vi "Overlay Pattern Matching Results #.vi"(7 "Group":string, 8 "error in":errorcluster, 9 "Result(PM)":cluster{"Name":string, "NG?":bool, "Score":dbl}, 10 "Matches":T2(array[cluster]), 11 "Image":T1) -> (0 "error out":errorcluster, 3 "Image Out":T1)   [LabVIEW 2013]
uses:
  <vilib>/vision/Image Controls.llb/IMAQ Image.ctl
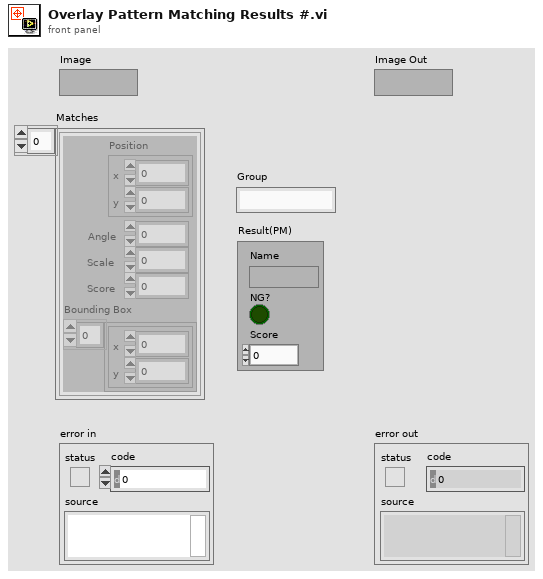
[diagram p1: front panel]
types:
  T1 = typedef "IMAQ Image.ctl" = refnum<image>
  T2 = cluster{"Position":cluster{"x":sgl, "y":sgl}, "Angle":sgl, "Scale":sgl, "Score":sgl, "Bounding Box":cluster{"x":sgl, "y":sgl}[]}[]
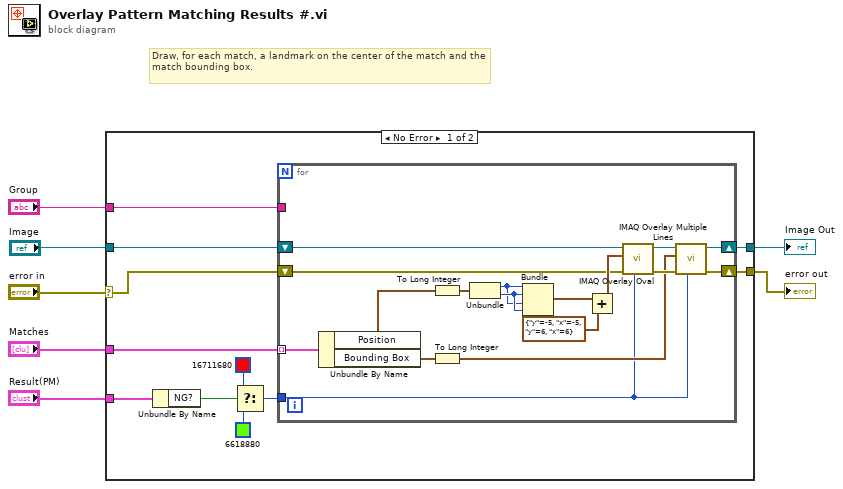
[diagram p0: block diagram]
diagram:
  # "Draw, for each match, a landmark on the center of the match and the match bounding box."
  n1 = case shown="No Error" "error in" {
    selector: "error in" -> [w13 w37]
    tunnel: "Matches" -> [w18 _]
    tunnel: [w17 w36] -> w6
    tunnel: "Image" -> [w16 w36]
    tunnel: [w15 w37] -> w4
    tunnel: "Group" -> [w14 _]
    tunnel: "Result(PM)" -> [w12 _]
    frame No Error {
      n2 = Unbundle By Name(w12) -> ("NG?"=w8:bool)
      n3 = Select(t=u32 16711680 ("Color"), s=w8, f=u32 6618880 ("Color")) -> (s? t:f=w9:u32)
      n4 = for {
        shift-right: [w23] -> w17
        shift-left: w16 -> [w22]
        tunnel: w18 -> [w35] mode=indexing
        tunnel: w9 -> [w19]
        shift-right: [w21] -> w15
        shift-left: w13 -> [w20]
        tunnel: w14 -> [_]
        n5 = Unbundle By Name(w35) -> ("Position"=w25:cluster{"x":sgl, "y":sgl}, "Bounding Box"=w24:cluster{"x":sgl, "y":sgl}[])
        n6 = To Long Integer(number=w25) -> (32bit integer=w31:cluster{"x":i32, "y":i32})
        n7 = To Long Integer(number=w24) -> (32bit integer=w32:cluster{"x":i32, "y":i32}[])
        n8 = Unbundle(w31) -> ("x"=w26:i32, "y"=w27:i32)
        n9 = Bundle("x"=w26, "y"=w27, "x"=w26, "y"=w27) -> (w28:cluster{"x":i32, "y":i32, "x":i32, "y":i32})  [unwired: 1 out]
        n10 = Add(x=w28, y=cluster{"y":i32, "x":i32, "y":i32, "x":i32} {"y"=-5, "x"=-5, "y"=6, "x"=6}) -> (x+y=w30:cluster{i32, i32, i32, i32})
        n11 = call "IMAQ Overlay Oval"("Color"=w19, "error in (no error)"=w20, "Bounding Rectangle"=w30, "Image"=w22) -> ("error out"=w33:errorcluster, "Image Out"=w34:T1)  [unwired: 2 in, 4 out]
        n12 = call "IMAQ Overlay Multiple Lines"("Color"=w19, "error in (no error)"=w33, "Line End Points"=w32, "Image"=w34) -> ("error out"=w21:errorcluster, "Image Out"=w23:T1)  [unwired: 2 in, 4 out]
      }
    }
    frame Error {
    }
  }
  "Image Out" <- w6
  "error out" <- w4
